vi "CalTxFrequency.vi"(0 "NI-RFSA Handle In":refnum<k15>, 1 "Enable PA":enum8{"0", "1"}(ring), 2 "Resp Timeout (ms)":i32 min=0, 3 "CW Freq (Hz)":i64=1, 4 "Active Dut":T2, 5 "Rx Central Frequency (Hz)":i64=1000000000, 7 "Rx Span (Hz)":dbl=192000.0 format="%.3p", 9 "FPGA Reference":refnum<k20>, 11 "error in (no error)":errorcluster, 12 "Freq Offset (Hz)":i64=1, 13 "Pwr Reduction (dB/2)":i8=1, 14 "CW Type":enum8{"0", "1", "2"}(ring)) -> (6 "Meas Power":dbl, 10 "Meas Frequency":dbl, 15 "error out":errorcluster)   [LabVIEW 2018]
uses:
  Resources_Test/UART/ControlTestSlot.ctl
  <vilib>/RFmx/RFInstr/mx/Support/RFmxInstrSupport.llb/niRFmx Instrument Handle.ctl
panel:
  in  "Instrument Handle In":T1
  out "Spectrum":cluster{"x0":dbl, "dx":dbl, "y":sgl[]}(graph)
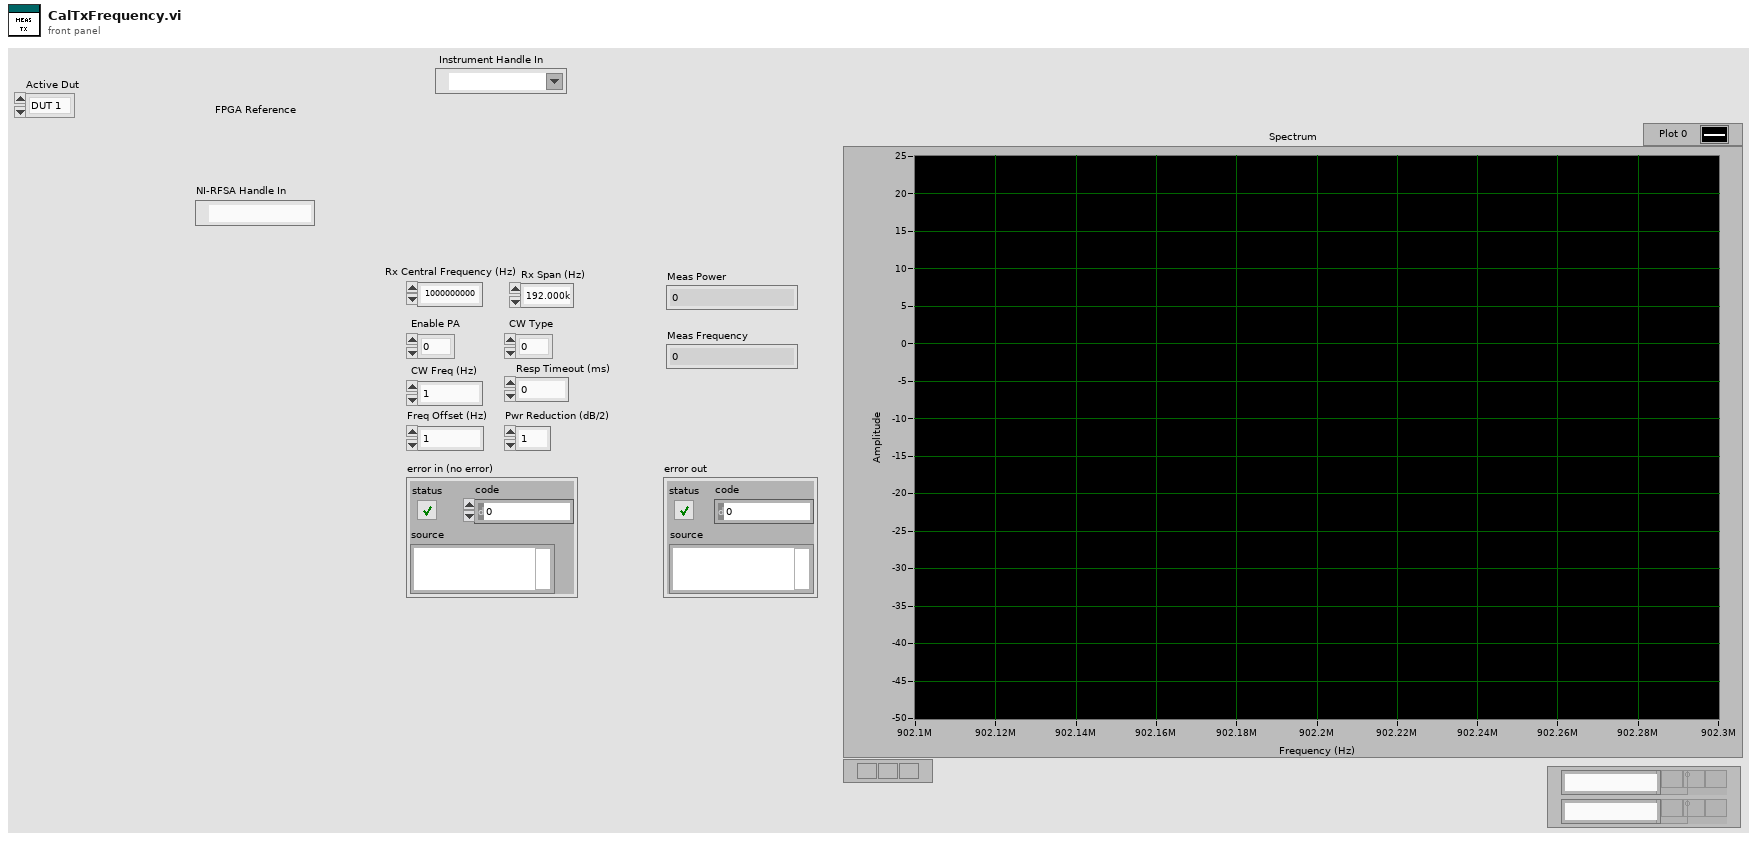
[diagram p1: front panel]
types:
  T1 = typedef "niRFmx Instrument Handle.ctl" = refnum<k21>
  T2 = typedef "ControlTestSlot.ctl" = enum16{"DUT 1", "DUT 2"}
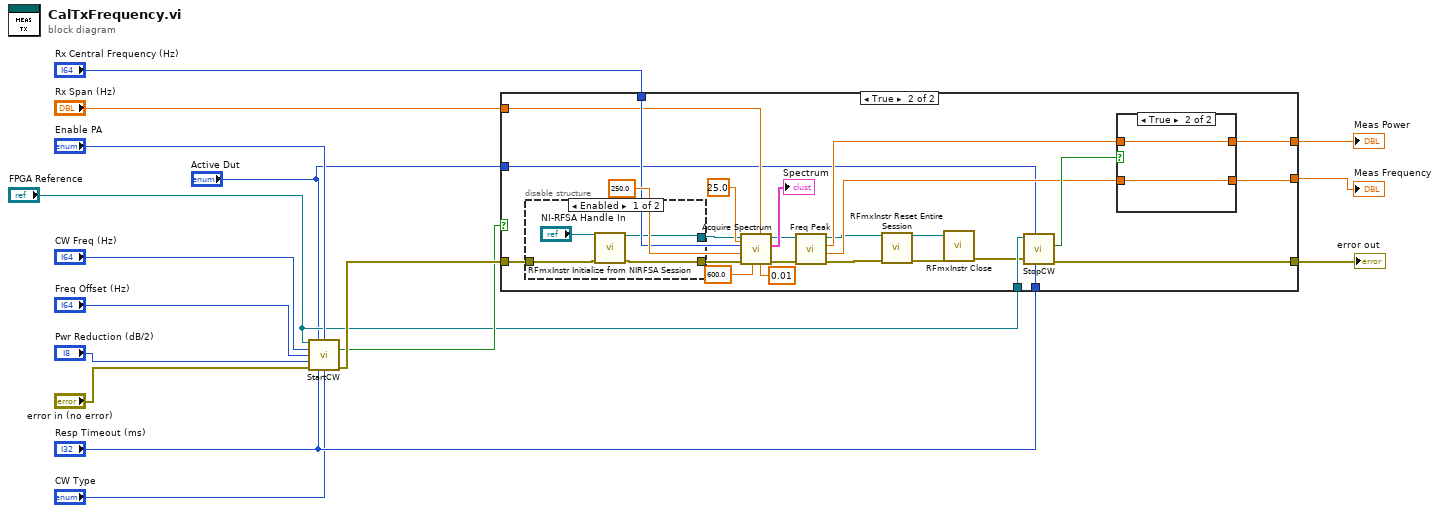
[diagram p0: block diagram]
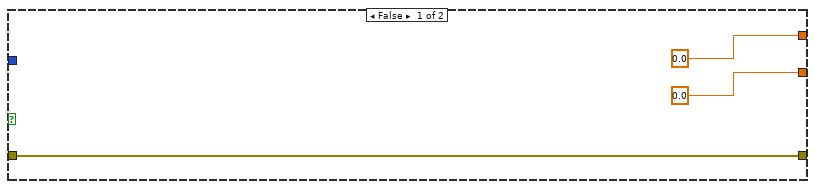
[diagram p2: hidden frame]
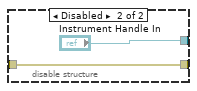
[diagram p3: hidden frame]
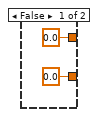
[diagram p4: hidden frame]
diagram:
  n1 = call "StartCW.vi"("FPGA Reference"="FPGA Reference", "Enum"="Active Dut", "Enable PA"="Enable PA", "CW Freq (Hz)"="CW Freq (Hz)", "Freq Offset (Hz)"="Freq Offset (Hz)", "Pwr Reduction (dB/2)"="Pwr Reduction (dB/2)", "Error In"="error in (no error)", "Resp Timeout (ms)"="Resp Timeout (ms)", "CW Type"="CW Type") -> ("Start CW OK"=w3:bool, "Error Out"=w4:errorcluster)  [unwired: 4 in, 1 out]
  n2 = case shown="True" w3 {
    tunnel: w4 -> [w19 w40]
    tunnel: "Rx Central Frequency (Hz)" -> [_ w37]
    tunnel: "Rx Span (Hz)" -> [_ w36]
    tunnel: "Resp Timeout (ms)" -> [_ w35]
    tunnel: [0.0 ("Peak Amplitude") w32] -> w14
    tunnel: [0.0 ("Peak Frequency (Hz)") w30] -> w13
    tunnel: [w19 w27] -> w12
    tunnel: "FPGA Reference" -> [_ w26]
    tunnel: "Active Dut" -> [_ w25]
    frame False {
    }
    frame True {
      n3 = disable-structure shown="Enabled" {
        disable-tunnel: w40 -> [w49 w51]
        disable-tunnel: [w48 w51] -> w39
        disable-tunnel: [w47 "Instrument Handle In"] -> w38
        frame Enabled {
          n4 = call <vilib>:"RFmxInstr Initialize from NIRFSA Session.vi"("NI-RFSA Handle In"="NI-RFSA Handle In", "error in (no error)"=w49) -> ("NI-RFmx Handle Out"=w47:refnum<k21>, "error out"=w48:errorcluster)  [unwired: 12 in]
        }
        frame Disabled {
        }
      }
      n5 = call "Acquire Spectrum.vi"("Acquisition Time (s)"=0.01, "Span (Hz)"=w36, "Sample Rate (S/s)"=600.0, "Reference Level"=25.0 ("reference level (dBm)"), "error in (no error)"=w39, "RBW (Hz)"=250.0 ("resolution bandwidth (Hz)"), "Center Frequency (Hz)"=w37, "Instrument Handle In"=w38) -> ("error out"=w43:errorcluster, "Spectrum"=→"Spectrum":cluster{"x0":dbl, "dx":dbl, "y":sgl[]}, "Instrument Handle Out"=w44:refnum<k21>)  [unwired: 1 in]
      n6 = call "Freq Peak.vi"("error in (no error)"=w43, "Instrument Handle In"=w44) -> ("error out"=w24:errorcluster, "Peak Frequency (Hz)"=w31:dbl, "Peak Amplitude"=w33:dbl, "Instrument Handle Out"=w23:refnum<k21>)  [unwired: 6 in]
      n7 = call <vilib>:"RFmxInstr Reset Entire Session.vi"("Instrument Handle In"=w23, "error in (no error)"=w24) -> ("Instrument Handle Out"=w22:refnum<k21>, "error out"=w21:errorcluster)  [unwired: 12 in]
      n8 = call <vilib>:"RFmxInstr Close.vi"("Instrument Handle In"=w22, "error in (no error)"=w21) -> ("error out"=w20:errorcluster)  [unwired: 13 in]
      n9 = call "StopCW.vi"("Resp Timeout (ms)"=w35, "Enum"=w25, "Error In"=w20, "FPGA Reference"=w26) -> ("Error Out"=w27:errorcluster, "Stop CW OK"=w34:bool)  [unwired: 5 in, 1 out]
      n10 = case shown="True" w34 {
        tunnel: w33 -> [_ w55]
        tunnel: [0.0 ("Peak Amplitude") w55] -> w32
        tunnel: w31 -> [_ w54]
        tunnel: [0.0 ("Peak Frequency (Hz)") w54] -> w30
        frame False {
        }
        frame True {
        }
      }
    }
  }
  "Meas Frequency" <- w13
  "Meas Power" <- w14
  "error out" <- w12
